vi "數字轉顏色.vi"(3 "數字":dbl) -> (1 "顏色數字":dbl)   [LabVIEW 2014]
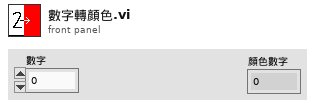
[diagram p1: front panel]
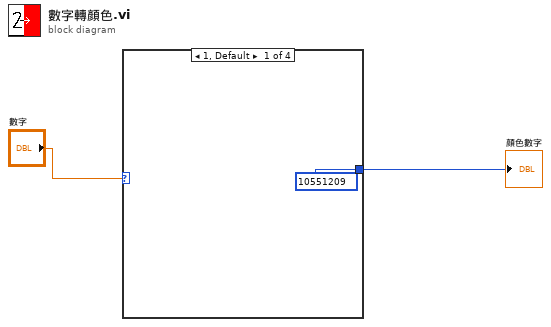
[diagram p0: block diagram]
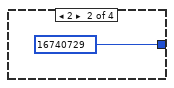
[diagram p2: hidden frame]
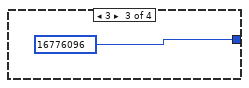
[diagram p3: hidden frame]
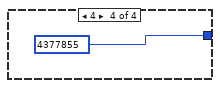
[diagram p4: hidden frame]
diagram:
  n1 = case shown="1, Default" "數字" {
    tunnel: [10551209 16740729 16776096 4377855] -> w1
    frame 1, Default {
    }
    frame 2 {
    }
    frame 3 {
    }
    frame 4 {
    }
  }
  "顏色數字" <- w1
